vi "pwmTest_wMotorController.vi"() -> ()   [LabVIEW 2017]
panel:
  in  "DutyCycle":dbl(slide) scale=0.0..100.0
  # "24v (100%)"
  # "0v (0%)"
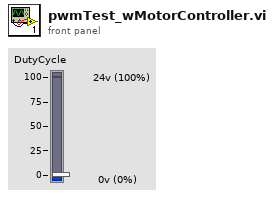
[diagram p1: front panel]
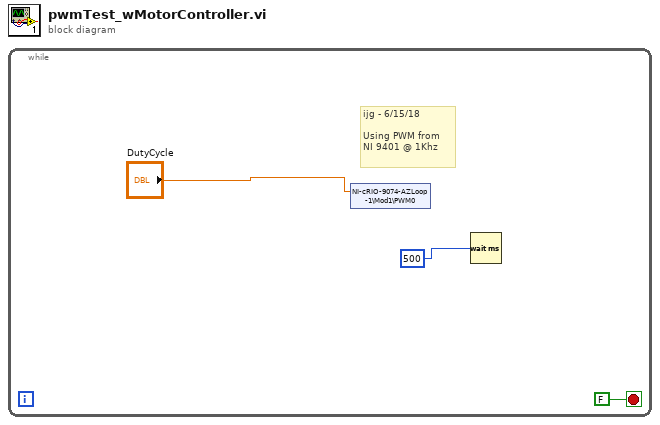
[diagram p0: block diagram]
diagram:
  n1 = while {
    stop <- FALSE stop-if-true
    # "ijg - 6/15/18\n\nUsing PWM from\nNI 9401 @ 1Khz"
    n2 = shared-variable "NI-cRIO-9074-AZLoop-1\\Mod1\\PWM0"("DutyCycle") -> ()  [unwired: 1 in, 1 out]
    n3 = Wait (ms)(milliseconds to wait=u32 500 ("millisecond multiple")) -> ()  [unwired: 1 out]
  }
